vi "Enable Output.vi"(8 "error in (no error)":errorcluster, 10 "Output On/off":bool, 11 "ARS-0220 in":refnum<class "ARS-0220.lvclass">) -> (0 "error out":errorcluster, 3 "ARS-0220 out":refnum<class "ARS-0220.lvclass">)   [LabVIEW 2016, in "Environment Chamber.lvlib" / "ARS-0220.lvclass"]
uses:
  ARS-0220.lvclass
  ARS-0220.lvclass/ARS-0220.ctl
  Support Libraries/Climatic Chamber/Climatic Chamber.lvlib
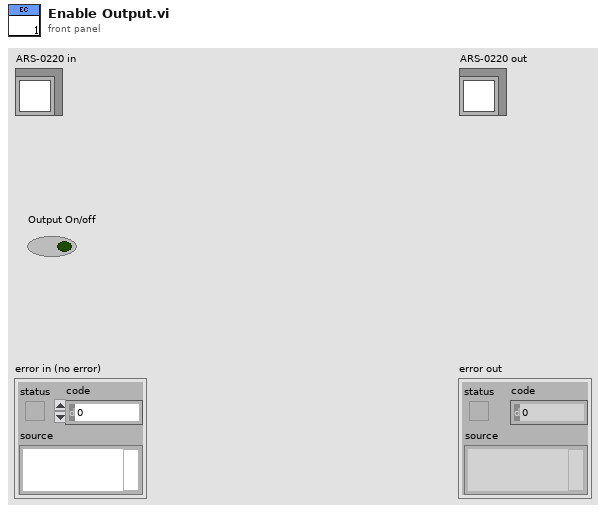
[diagram p1: front panel]
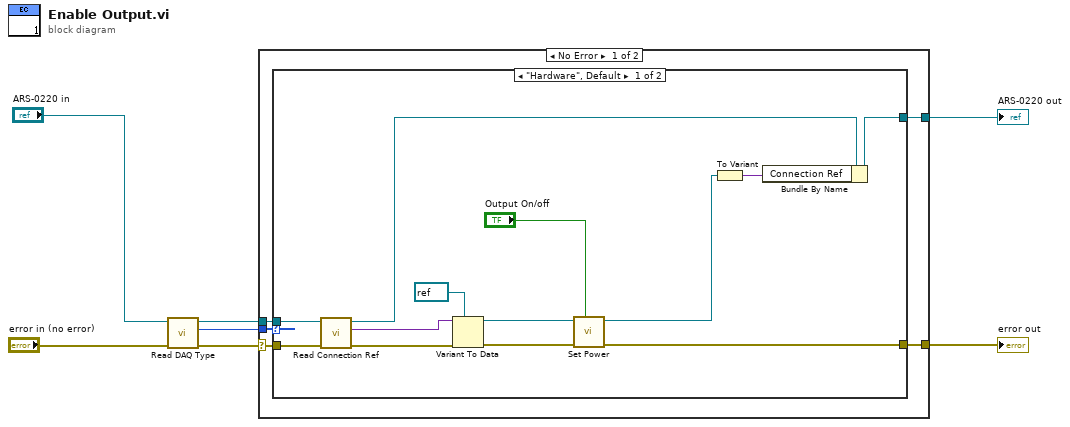
[diagram p0: block diagram]
diagram:
  n1 = call "Read DAQ Type.vi"("error in (no error)"="error in (no error)", "ARS-0220 in"="ARS-0220 in") -> ("error out"=w6:errorcluster, "DAQ Type"=w5:enum16{"Hardware", "Simulation"}, "ARS-0220 out"=w4:refnum<class "ARS-0220.lvclass">)  [unwired: 7 in]
  n2 = case shown="No Error" w6 {
    selector: w6 -> [w11 w29]
    tunnel: w5 -> [w12 _]
    tunnel: w4 -> [w10 w28]
    tunnel: [w9 w28] -> w2
    tunnel: [w8 w29] -> w1
    frame No Error {
      n3 = case shown="\"Hardware\", Default" w12 {
        tunnel: w11 -> [w25 w27]
        tunnel: w10 -> [w24 w26]
        tunnel: [w17 w26] -> w9
        tunnel: [w18 w27] -> w8
        frame "Hardware", Default {
          n4 = call "Read Connection Ref.vi"("error in (no error)"=w25, "ARS-0220 in"=w24) -> ("error out"=w23:errorcluster, "Connection Ref"=w22:variant, "ARS-0220 out"=w14:refnum<class "ARS-0220.lvclass">)  [unwired: 7 in]
          n5 = Variant To Data(error in=w23, type=refnum<visa-resource-name> refnum ("VISA resource name"), Variant=w22) -> (data=w19:refnum<visa-resource-name>, error out=w20:errorcluster)
          n6 = call "Set Power.vi"("Power (On/Off)"="Output On/off", "error in (no error)"=w20, "VISA resource name"=w19) -> ("error out"=w18:errorcluster, "VISA resource name out"=w15:refnum<visa-resource-name>)  [unwired: 7 in]
          n7 = To Variant(anything=w15) -> (Variant=w16:variant)
          n8 = Bundle By Name(cluster=w14, "Connection Ref"=w16) -> (w17:refnum<class "ARS-0220.lvclass">)
        }
        frame "Simulation" {
        }
      }
    }
    frame Error {
    }
  }
  "error out" <- w1
  "ARS-0220 out" <- w2
